vi "LEDSA --ALL IO--.vi"(2 "Error In 2":errorcluster, 3 "FPGA VI Reference In":T1) -> (0 "Error Out 2":errorcluster, 1 "FPGA VI Reference Out":T2)   [LabVIEW 2015]
uses:
  FPGA Ref Out.ctl
  FPGA Ref In.ctl
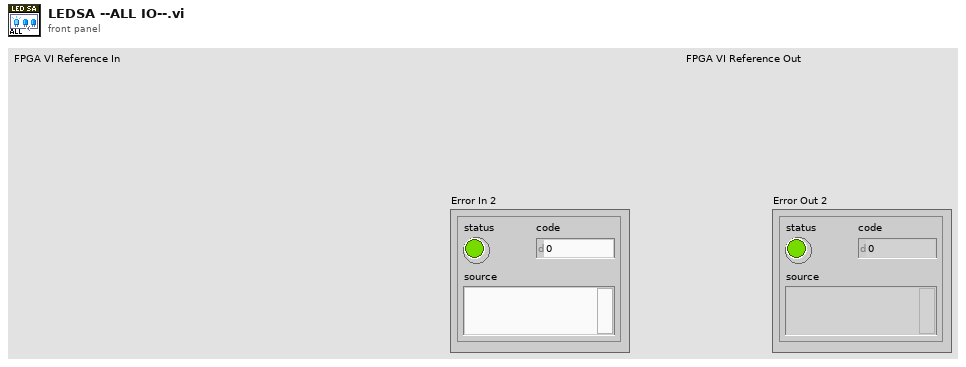
[diagram p1: front panel]
types:
  T1 = typedef "FPGA Ref In.ctl" = refnum<k20>
  T2 = typedef "FPGA Ref Out.ctl" = refnum<k20>
  T3 = cluster{"LED 3":enum16{"Brightness", "Bool"}, "BOOL":bool, "Brightness":u32}
  T4 = cluster{"LED 1":enum16{"Brightness", "Bool"}, "BOOL":bool, "Brightness":u32}
  T5 = cluster{"LED 2":enum16{"Brightness", "Bool"}, "BOOL":bool, "Brightness":u32}
  T6 = cluster{"LED 0":enum16{"Brightness", "Bool"}, "BOOL":bool, "Brightness":u32}
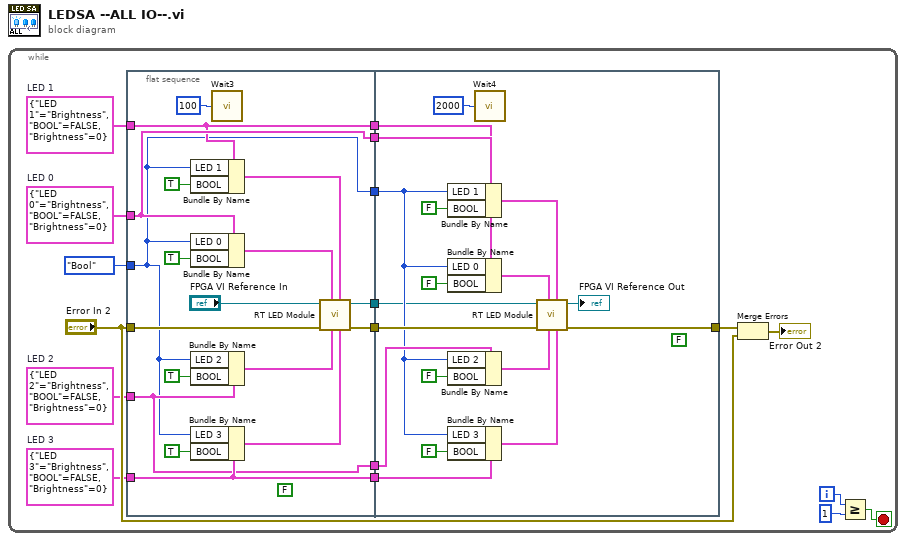
[diagram p0: block diagram]
diagram:
  n1 = while {
    i -> [w14]
    stop <- w12 stop-if-true
    w6 = T3 {"LED 3"=enum."Brightness", "BOOL"=FALSE, "Brightness"=0}  # LED 3
    w4 = T4 {"LED 1"=enum."Brightness", "BOOL"=FALSE, "Brightness"=0}  # LED 1
    w5 = T5 {"LED 2"=enum."Brightness", "BOOL"=FALSE, "Brightness"=0}  # LED 2
    w11 = T6 {"LED 0"=enum."Brightness", "BOOL"=FALSE, "Brightness"=0}  # LED 0
    n2 = flat-sequence {
      tunnel: "Error In 2" -> [w35]
      tunnel: [w34] -> w18
      tunnel: w11 -> [w33]
      tunnel: [w33] -> w10
      tunnel: [w32] -> w9
      tunnel: [w31] -> w8
      tunnel: [w30] -> w7
      tunnel: w6 -> [w32]
      tunnel: w5 -> [w31]
      tunnel: w4 -> [w30]
      tunnel: enum16{"Brightness", "Bool"}."Bool" ("LED") -> [w29]
      tunnel: [w29] -> w2
      tunnel: [w20] -> w1
      tunnel: w18 -> [w53]
      tunnel: [w52] -> w17
      tunnel: w10 -> [w51]
      tunnel: w9 -> [w50]
      tunnel: w8 -> [w49]
      tunnel: w7 -> [w48]
      tunnel: w2 -> [w47]
      tunnel: w1 -> [w38]
      frame #0 {
        (unwired) FALSE ("Stop Button")
        n3 = Bundle By Name(cluster=w30, "LED 1"=w29, "BOOL"=TRUE ("LED 1")) -> (w23:T4)
        n4 = Bundle By Name(cluster=w33, "LED 0"=w29, "BOOL"=TRUE ("LED 0")) -> (w24:T6)
        n5 = Bundle By Name(cluster=w31, "LED 2"=w29, "BOOL"=TRUE ("LED 2")) -> (w22:T5)
        n6 = Bundle By Name(cluster=w32, "LED 3"=w29, "BOOL"=TRUE ("LED 3")) -> (w21:T3)
        n7 = call "Wait3"("Count(mSec)"=u32 100) -> ()  [unwired: 1 out]
        n8 = call "RT LED Module.vi"("LED 3"=w21, "LED 1"=w23, "LED 2"=w22, "LED 0"=w24, "error in"=w35, "FPGA VI Reference In"="FPGA VI Reference In") -> ("error out"=w34:errorcluster, "FPGA VI Reference Out"=w20:T2)  [unwired: 4 in]
      }
      frame #1 {
        (unwired) FALSE ("Stop Button")
        n9 = Bundle By Name(cluster=w48, "LED 1"=w47, "BOOL"=FALSE ("LED 2")) -> (w41:T4)
        n10 = Bundle By Name(cluster=w51, "LED 0"=w47, "BOOL"=FALSE ("LED 3")) -> (w42:T6)
        n11 = Bundle By Name(cluster=w49, "LED 2"=w47, "BOOL"=FALSE ("LED 0")) -> (w40:T5)
        n12 = Bundle By Name(cluster=w50, "LED 3"=w47, "BOOL"=FALSE ("LED 1")) -> (w39:T3)
        n13 = call "Wait4"("Count(mSec)"=u32 2000) -> ()  [unwired: 1 out]
        n14 = call "RT LED Module.vi"("LED 3"=w39, "LED 1"=w41, "LED 2"=w40, "LED 0"=w42, "error in"=w53, "FPGA VI Reference In"=w38) -> ("error out"=w52:errorcluster, "FPGA VI Reference Out"=→"FPGA VI Reference Out":T2)  [unwired: 4 in]
      }
    }
    n15 = Merge Errors(w17, "Error In 2") -> (→"Error Out 2":errorcluster)
    n16 = Greater Or Equal?(x=w14, y=1) -> (x >= y?=w12:bool)
  }
